vi "rsidr_core_global.vi"() -> ()   [LabVIEW 2020, in "Rohde&Schwarz RTx Oscilloscopes.lvlib"] (continued)
 is white. You can select another monochrome color, or a color scale.\n\nAvailable Repeated Capabilities:\nReferenceWfm: RW1, RW2, RW3, RW4\r\n\nRemote-control command(s):\nREFCurve<m>:WCOLor"}, {"Level"=2, "Class Only"=TRUE, "Identifier"="", "Descriptive Name"="Reference", "Data Type"=0, "Command"="", "Access"=0, "Range Table"="", "Read Callback"="", "Write Callback"="", "Supported Models"="", "Instrument Options"="", "Flags"=0, "Help"="Contains attributes for Reference settings."}, {"Level"=3, "Class Only"=FALSE, "Identifier"="RSRTX_ATTR_REFERENCE_WAVEFORM_SOURCE", "Descriptive Name"="Reference Waveform Source", "Data Type"=0, "Command"="REFC{ReferenceWfm}:SOUR", "Access"=2, "Range Table"="rsrtx_rngReferenceWaveformParameter", "Read Callback"="", "Write Callback"="", "Supported Models"="", "Instrument Options"="", "Flags"=0, "Help"="Selects the source waveform to be used as a reference.\n\nAvailable Repeated Capabilities:\nReferenceWfm: RW1, RW2, RW3, RW4\r\n\nRemote-control command(s):\nREFCurve<m>:SOURce"}, {"Level"=3, "Class Only"=FALSE, "Identifier"="RSRTX_ATTR_REFERENCE_WAVEFORM_UPDATE", "Descriptive Name"="Reference Waveform Update", "Data Type"=4, "Command"="REFC{ReferenceWfm}:UPD", "Access"=1, "Range Table"="", "Read Callback"="", "Write Callback"="", "Supported Models"="", "Instrument Options"="", "Flags"=0, "Help"="Copies the selected source waveform with all its settings to the memory of the reference waveform\n\nAvailable Repeated Capabilities:\nReferenceWfm: RW1, RW2, RW3, RW4\r\n\nRemote-control command(s):\nREFCurve<m>:UPDate"}, {"Level"=3, "Class Only"=FALSE, "Identifier"="RSRTX_ATTR_REFERENCE_WAVEFORM_DISPLAY_ENABLED", "Descriptive Name"="Reference Waveform Display Enabled", "Data Type"=3, "Command"="REFC{ReferenceWfm}:STAT", "Access"=2, "Range Table"="", "Read Callback"="", "Write Callback"="", "Supported Models"="", "Instrument Options"="", "Flags"=0, "Help"="If enabled, the reference waveform is displayed in the diagram.\n\nAvailable Repeated Capabilities:\nReferenceWfm: RW1, RW2, RW3, RW4\r\n\nRemote-control command(s):\nREFCurve<m>:STATe"}, {"Level"=3, "Class Only"=FALSE, "Identifier"="RSRTX_ATTR_REFERENCE_WAVEFORM_LOAD_FROM_FILE", "Descriptive Name"="Reference Waveform Load From File", "Data Type"=2, "Command"="REFC{ReferenceWfm}:LOAD", "Access"=1, "Range Table"="", "Read Callback"="", "Write Callback"="", "Supported Models"="", "Instrument Options"="", "Flags"=0, "Help"="Loads the waveform data from the indicated reference file to the reference storage. To load the instrument settings, use REFCurve<m>: LOAD: STATe.\n\nAvailable Repeated Capabilities:\nReferenceWfm: RW1, RW2, RW3, RW4\r\n\nRemote-control command(s):\nREFCurve<m>:LOAD"}, {"Level"=3, "Class Only"=FALSE, "Identifier"="RSRTX_ATTR_REFERENCE_WAVEFORM_LOAD_CONFIGURATION", "Descriptive Name"="Reference Waveform Load Configuration", "Data Type"=4, "Command"="REFC{ReferenceWfm}:LOAD:STAT", "Access"=1, "Range Table"="", "Read Callback"="", "Write Callback"="", "Supported Models"="", "Instrument Options"="", "Flags"=0, "Help"="Loads the instrument settings in addition to the reference waveform data. The waveform data must be loaded before the settings. The settings are only available if the file was stored to the internal storage /INT/REF ERENCE and never written to an external storage (USB stick).\n\nAvailable Repeated Capabilities:\nReferenceWfm: RW1, RW2, RW3, RW4\r\n\nRemote-control command(s):\nREFCurve<m>:LOAD:STATe"}, {"Level"=3, "Class Only"=FALSE, "Identifier"="RSRTX_ATTR_REFERENCE_WAVEFORM_SAVE_TO_FILE", "Descriptive Name"="Reference Waveform Save To File", "Data Type"=2, "Command"="REFC{ReferenceWfm}:SAVE", "Access"=1, "Range Table"="", "Read Callback"="", "Write Callback"="", "Supported Models"="", "Instrument Options"="", "Flags"=0, "Help"="Stores the reference waveform the specified file. For instrument model &apos;&apos; is parameter <FileName> ignored.\n\nAvailable Repeated Capabilities:\nReferenceWfm: RW1, RW2, RW3, RW4\r\n\nRemote-control command(s):\nREFCurve<m>:SAVE"}, {"Level"=3, "Class Only"=FALSE, "Identifier"="RSRTX_ATTR_REFERENCE_WAVEFORM_CATALOG", "Descriptive Name"="Reference Waveform Catalog", "Data Type"=2, "Command"="REFC{ReferenceWfm}:SOUR:CAT?", "Access"=0, "Range Table"="", "Read Callback"="", "Write Callback"="", "Supported Models"="", "Instrument Options"="", "Flags"=0, "Help"="Returns the source waveform - channel, math or reference waveform.\n\nAvailable Repeated Capabilities:\nReferenceWfm: RW1, RW2, RW3, RW4\r\n\nRemote-control command(s):\nREFCurve<m>:SOURce:CATalog?"}, {"Level"=2, "Class Only"=TRUE, "Identifier"="", "Descriptive Name"="Scaling", "Data Type"=0, "Command"="", "Access"=0, "Range Table"="", "Read Callback"="", "Write Callback"="", "Supported Models"="", "Instrument Options"="", "Flags"=0, "Help"="Contains attributes for Scalling settings."}, {"Level"=3, "Class Only"=FALSE, "Identifier"="RSRTX_ATTR_REFERENCE_WAVEFORM_VERTICAL_SCALE", "Descriptive Name"="Reference Waveform Vertical Scale", "Data Type"=1, "Command"="REFC{ReferenceWfm}:VERT:SCAL", "Access"=2, "Range Table"="", "Read Callback"="", "Write Callback"="", "Supported Models"="", "Instrument Options"="", "Flags"=0, "Help"="Sets the scale factor for the reference waveform if vertical scaling is set to Independent.\n\nAvailable Repeated Capabilities:\nReferenceWfm: RW1, RW2, RW3, RW4\r\n\nRemote-control command(s):\nREFCurve<m>:VERTical:SCALe"}, {"Level"=3, "Class Only"=FALSE, "Identifier"="RSRTX_ATTR_REFERENCE_WAVEFORM_VERTICAL_POSITION", "Descriptive Name"="Reference Waveform Vertical Position", "Data Type"=1, "Command"="REFC{ReferenceWfm}:VERT:POS", "Access"=2, "Range Table"="", "Read Callback"="", "Write Callback"="", "Supported Models"="", "Instrument Options"="", "Flags"=0, "Help"="Moves the reference waveform and its horizontal axis up or down in the diagram, if vertical scaling is set to Independent.\n\nAvailable Repeated Capabilities:\nReferenceWfm: RW1, RW2, RW3, RW4\r\n\nRemote-control command(s):\nREFCurve<m>:VERTical:POSition"}, {"Level"=3, "Class Only"=FALSE, "Identifier"="RSRTX_ATTR_REFERENCE_WAVEFORM_HORIZONTAL_SCALE", "Descriptive Name"="Reference Waveform Horizontal Scale", "Data Type"=1, "Command"="REFC{ReferenceWfm}:HOR:SCAL", "Access"=2, "Range Table"="", "Read Callback"="", "Write Callback"="", "Supported Models"="", "Instrument Options"="", "Flags"=0, "Help"="Changes the horizontal scale (timebase) of the reference waveform independent of the channel waveform settings.\n\nAvailable Repeated Capabilities:\nReferenceWfm: RW1, RW2, RW3, RW4\r\n\nRemote-control command(s):\nREFCurve<m>:HORizontal:SCALe"}, {"Level"=3, "Class Only"=FALSE, "Identifier"="RSRTX_ATTR_REFERENCE_WAVEFORM_HORIZONTAL_POSITION", "Descriptive Name"="Reference Waveform Horizontal Position", "Data Type"=1, "Command"="REFC{ReferenceWfm}:HOR:POS", "Access"=2, "Range Table"="", "Read Callback"="", "Write Callback"="", "Supported Models"="", "Instrument Options"="", "Flags"=0, "Help"="Changes the horizontal position of the reference waveform independent of the channel waveform settings.\n\nAvailable Repeated Capabilities:\nReferenceWfm: RW1, RW2, RW3, RW4\r\n\nRemote-control command(s):\nREFCurve<m>:HORizontal:POSition"}, {"Level"=1, "Class Only"=TRUE, "Identifier"="", "Descriptive Name"="Mask", "Data Type"=0, "Command"="", "Access"=0, "Range Table"="", "Read Callback"="", "Write Callback"="", "Supported Models"="", "Instrument Options"="", "Flags"=0, "Help"="Contains attributes for Masks settings."}, {"Level"=2, "Class Only"=FALSE, "Identifier"="RSRTX_ATTR_MASK_ENABLED", "Descriptive Name"="Mask Enabled", "Data Type"=3, "Command"="MASK:STAT", "Access"=2, "Range Table"="", "Read Callback"="", "Write Callback"="", "Supported Models"="", "Instrument Options"="", "Flags"=0, "Help"="Turns the mask test mode on or off. When turning off, any temporarily stored new masks are deleted.\n\nAvailable Repeated Capabilities:\nNone\n\nRemote-control command(s):\nMASK:STATe"}, {"Level"=2, "Class Only"=FALSE, "Identifier"="RSRTX_ATTR_MASK_SOURCE", "Descriptive Name"="Mask Source", "Data Type"=0, "Command"="MASK:SOUR", "Access"=2, "Range Table"="rsrtx_rngSource", "Read Callback"="", "Write Callback"="", "Supported Models"="", "Instrument Options"="", "Flags"=0, "Help"="Defines the channel to be compared with the mask.\n\nAvailable Repeated Capabilities:\nNone\n\nRemote-control command(s):\nMASK:SOURce"}, {"Level"=2, "Class Only"=FALSE, "Identifier"="RSRTX_ATTR_MASK_TEST", "Descriptive Name"="Mask Test", "Data Type"=0, "Command"="MASK:TEST", "Access"=2, "Range Table"="rsrtx_rngMaskCondition", "Read Callback"="", "Write Callback"="", "Supported Models"="", "Instrument Options"="", "Flags"=0, "Help"="Starts, finishes or interrupts a mask test.\n\nAvailable Repeated Capabilities:\nNone\n\nRemote-control command(s):\nMASK:TEST"}, {"Level"=2, "Class Only"=FALSE, "Identifier"="RSRTX_ATTR_MASK_COPY_CHANNEL", "Descriptive Name"="Mask Copy Channel", "Data Type"=4, "Command"="MASK:CHC", "Access"=1, "Range Table"="", "Read Callback"="", "Write Callback"="", "Supported Models"="", "Instrument Options"="", "Flags"=0, "Help"="Creates a mask from the envelope waveform of the test source set with MASK:SOURce.\n\nAvailable Repeated Capabilities:\nNone\n\nRemote-control command(s):\nMASK:CHCopy"}, {"Level"=2, "Class Only"=FALSE, "Identifier"="RSRTX_ATTR_MASK_HIT_COUNT", "Descriptive Name"="Mask Hit Count", "Data Type"=0, "Command"="MASK:VCO?", "Access"=0, "Range Table"="", "Read Callback"="", "Write Callback"="", "Supported Models"="", "Instrument Options"="", "Flags"=0, "Help"="Returns the number of acquistions that hit the mask.\n\nAvailable Repeated Capabilities:\nNone\n\nRemote-control command(s):\nMASK:VCOunt?"}, {"Level"=2, "Class Only"=FALSE, "Identifier"="RSRTX_ATTR_MASK_COUNT", "Descriptive Name"="Mask Count", "Data Type"=0, "Command"="MASK:COUN?", "Access"=0, "Range Table"="", "Read Callback"="", "Write Callback"="", "Supported Models"="", "Instrument Options"="", "Flags"=0, "Help"="Returns the number of tested acquisitions.\n\nAvailable Repeated Capabilities:\nNone\n\nRemote-control command(s):\nMASK:COUNt?"}, {"Level"=2, "Class Only"=FALSE, "Identifier"="RSRTX_ATTR_MASK_SEGMENT_CAPTURE_MODE", "Descriptive Name"="Mask Segment Capture Mode", "Data Type"=0, "Command"="MASK:CAPT", "Access"=2, "Range Table"="RsRtx_rngMaskCaptureMode", "Read Callback"="", "Write Callback"="", "Supported Models"="", "Instrument Options"="K15", "Flags"=0, "Help"="Only available with history. Selects whether all acquisitions are stored in segments, or only failed acquisition. You can use the history to analyze the segments.\n\nAvailable Repeated Capabilities:\nNone\n\nRemote-control command(s):\nMASK:CAPTure[:MODE]"}, {"Level"=2, "Class Only"=FALSE, "Identifier"="RSRTX_ATTR_MASK_STORE", "Descriptive Name"="Mask Store", "Data Type"=2, "Command"="MASK:SAVE", "Access"=1, "Range Table"="", "Read Callback"="", "Write Callback"="", "Supported Models"="", "Instrument Options"="", "Flags"=0, "Help"="Saves the current mask in the specified file.\n\nAvailable Repeated Capabilities:\nNone\n\nRemote-control command(s):\nMASK:SAVE"}, {"Level"=2, "Class Only"=FALSE, "Identifier"="RSRTX_ATTR_MASK_LOAD", "Descriptive Name"="Mask Load", "Data Type"=2, "Command"="MASK:LOAD", "Access"=1, "Range Table"="", "Read Callback"="", "Write Callback"="", "Supported Models"="", "Instrument Options"="", "Flags"=0, "Help"="Loads a stored mask from the specified file.\n\nAvailable Repeated Capabilities:\nNone\n\nRemote-control command(s):\nMASK:LOAD"}, {"Level"=2, "Class Only"=FALSE, "Identifier"="RSRTX_ATTR_MASK_TEST_ACTION_BEEP", "Descriptive Name"="Mask Test Action Beep", "Data Type"=0, "Command"="MASK:ACT:SOUN:EVEN:MODE", "Access"=2, "Range Table"="rsrtx_rngMaskTestActionExecution", "Read Callback"="", "Write Callback"="", "Supported Models"="", "Instrument Options"="", "Flags"=0, "Help"="Sets when and how often the generates a beep sound will be executed.\n\nAvailable Repeated Capabilities:\nNone\n\nRemote-control command(s):\nMASK:ACTion:SOUNd:EVENt:MODE"}, {"Level"=2, "Class Only"=FALSE, "Identifier"="RSRTX_ATTR_MASK_TEST_ACTION_STOP", "Descriptive Name"="Mask Test Action Stop", "Data Type"=0, "Command"="MASK:ACT:STOP:EVEN:MODE", "Access"=2, "Range Table"="rsrtx_rngMaskTestActionExecution", "Read Callback"="", "Write Callback"="", "Supported Models"="", "Instrument Options"="", "Flags"=0, "Help"="Sets when and how often the stops the waveform acquisition. will be executed.\n\nAvailable Repeated Capabilities:\nNone\n\nRemote-control command(s):\nMASK:ACTion:STOP:EVENt:MODE"}, {"Level"=2, "Class Only"=FALSE, "Identifier"="RSRTX_ATTR_MASK_TEST_ACTION_SCREENSHOT", "Descriptive Name"="Mask Test Action Screenshot", "Data Type"=0, "Command"="MASK:ACT:SCRS:EVEN:MODE", "Access"=2, "Range Table"="rsrtx_rngMaskTestActionExecution", "Read Callback"="", "Write Callback"="", "Supported Models"="", "Instrument Options"="", "Flags"=0, "Help"="Sets when and how often the saves a screenshot according to printer output settings will be executed.\n\nAvailable Repeated Capabilities:\nNone\n\nRemote-control command(s):\nMASK:ACTion:SCRSave:EVENt:MODE"}, {"Level"=2, "Class Only"=FALSE, "Identifier"="RSRTX_ATTR_MASK_TEST_ACTION_SCREENSHOT_DESTINATION", "Descriptive Name"="Mask Test Action Screenshot Destination", "Data Type"=2, "Command"="MASK:ACT:SCRS:DEST", "Access"=2, "Range Table"="", "Read Callback"="", "Write Callback"="", "Supported Models"="", "Instrument Options"="", "Flags"=0, "Help"="Defines the path and filename for a screenshot that will be saved on mask violation. The file format is PNG, the filename is incremented automatically.\n\nAvailable Repeated Capabilities:\nNone\n\nRemote-control command(s):\nMASK:ACTion:SCRSave:DESTination"}, {"Level"=2, "Class Only"=FALSE, "Identifier"="RSRTX_ATTR_MASK_TEST_ACTION_SAVES_WAVEFORM", "Descriptive Name"="Mask Test Action Saves Waveform", "Data Type"=0, "Command"="MASK:ACT:WFMSave:EVEN:MODE", "Access"=2, "Range Table"="rsrtx_rngMaskTestActionExecution", "Read Callback"="", "Write Callback"="", "Supported Models"="", "Instrument Options"="", "Flags"=0, "Help"="Sets when and how often the saves the waveform data according to the screenshot output settings will be executed.\n\nAvailable Repeated Capabilities:\nNone\n\nRemote-control command(s):\nMASK:ACTion:WFMSave:EVENt:MODE"}, {"Level"=2, "Class Only"=FALSE, "Identifier"="RSRTX_ATTR_MASK_TEST_ACTION_SAVES_WAVEFORM_DESTINATION", "Descriptive Name"="Mask Test Action Saves Waveform Destination", "Data Type"=2, "Command"="MASK:ACT:WFMS:DEST", "Access"=2, "Range Table"="", "Read Callback"="", "Write Callback"="", "Supported Models"="", "Instrument Options"="", "Flags"=0, "Help"="Defines the path and filename for a waveform data that will be saved on mask violation. The file format is CSV, the filename is incremented automatically.\n\nAvailable Repeated Capabilities:\nNone\n\nRemote-control command(s):\nMASK:ACTion:WFMSave:DESTination"}, {"Level"=2, "Class Only"=FALSE, "Identifier"="RSRTX_ATTR_MASK_TEST_ACTION_PULSE", "Descriptive Name"="Mask Test Action Pulse", "Data Type"=0, "Command"="MASK:ACT:PULS:EVEN:MODE", "Access"=2, "Range Table"="rsrtx_rngMaskTestActionExecution", "Read Callback"="", "Write Callback"="", "Supported Models"="", "Instrument Options"="", "Flags"=0, "Help"="Creates a trigger out pulse on mask violation.\n\nAvailable Repeated Capabilities:\nNone\n\nRemote-control command(s):\nMASK:ACTion:PULSe:EVENt:MODE"}, {"Level"=2, "Class Only"=FALSE, "Identifier"="RSRTX_ATTR_MASK_TEST_ACTION_AUX_OUTPUT_ENABLED", "Descriptive Name"="Mask Test Action AUX Output Enabled", "Data Type"=3, "Command"="MASK:ACT:YOUT:ENAB", "Access"=2, "Range Table"="", "Read Callback"="", "Write Callback"="", "Supported Models"="", "Instrument Options"="", "Flags"=0, "Help"="Creates a pulse on the AUX OUT connector if the mask is violated. This selection sets the configuration of the AUX OUT connector to Mask Violation.\n\nAvailable Repeated Capabilities:\nNone\n\nRemote-control command(s):\nMASK:ACTion:YOUT:ENABle"}, {"Level"=2, "Class Only"=FALSE, "Identifier"="RSRTX_ATTR_MASK_TEST_VIOLATION_COUNT_BEEP", "Descriptive Name"="Mask Test Violation Count Beep", "Data Type"=0, "Command"="MASK:ACT:SOUN:EVEN:COUN", "Access"=2, "Range Table"="", "Read Callback"="", "Write Callback"="", "Supported Models"="", "Instrument Options"="", "Flags"=0, "Help"="Sets the number of mask violations after which the generates a beep sound is executed.\n\nAvailable Repeated Capabilities:\nNone\n\nRemote-control command(s):\nMASK:ACTion:SOUNd:EVENt:COUNt"}, {"Level"=2, "Class Only"=FALSE, "Identifier"="RSRTX_ATTR_MASK_TEST_VIOLATION_COUNT_STOP", "Descriptive Name"="Mask Test Violation Count Stop", "Data Type"=0, "Command"="MASK:ACT:STOP:EVEN:COUN", "Access"=2, "Range Table"="", "Read Callback"="", "Write Callback"="", "Supported Models"="", "Instrument Options"="", "Flags"=0, "Help"="Sets the number of mask violations after which the stops the waveform acquisition is executed.\n\nAvailable Repeated Capabilities:\nNone\n\nRemote-control command(s):\nMASK:ACTion:STOP:EVENt:COUNt"}, {"Level"=2, "Class Only"=FALSE, "Identifier"="RSRTX_ATTR_MASK_TEST_VIOLATION_COUNT_SCREENSHOT", "Descriptive Name"="Mask Test Violation Count Screenshot", "Data Type"=0, "Command"="MASK:ACT:SCRS:EVEN:COUN", "Access"=2, "Range Table"="", "Read Callback"="", "Write Callback"="", "Supported Models"="", "Instrument Options"="", "Flags"=0, "Help"="Sets the number of mask violations after which the saves a screenshot according to printer output settings is executed.\n\nAvailable Repeated Capabilities:\nNone\n\nRemote-control command(s):\nMASK:ACTion:SCRSave:EVENt:COUNt"}, {"Level"=2, "Class Only"=FALSE, "Identifier"="RSRTX_ATTR_MASK_TEST_VIOLATION_COUNT_PRINT", "Descriptive Name"="Mask Test Violation Count Print", "Data Type"=0, "Command"="MASK:ACT:PRIN:EVEN:COUN", "Access"=2, "Range Table"="", "Read Callback"="", "Write Callback"="", "Supported Models"="", "Instrument Options"="", "Flags"=0, "Help"="Sets the number of mask violations after which the prints a screenshot to a printer connected to the USB connector on the front or rear panel is executed.\n\nAvailable Repeated Capabilities:\nNone\n\nRemote-control command(s):\nMASK:ACTion:PRINt:EVENt:COUNt"}, {"Level"=2, "Class Only"=FALSE, "Identifier"="RSRTX_ATTR_MASK_TEST_VIOLATION_COUNT_SAVES_WAVEFORM", "Descriptive Name"="Mask Test Violation Count Saves Waveform", "Data Type"=0, "Command"="MASK:ACT:WFMS:EVEN:COUN", "Access"=2, "Range Table"="", "Read Callback"="", "Write Callback"="", "Supported Models"="", "Instrument Options"="", "Flags"=0, "Help"="Sets the number of mask violations after which the saves the waveform data according to the screenshot output settings is executed.\n\nAvailable Repeated Capabilities:\nNone\n\nRemote-control command(s):\nMASK:ACTion:WFMSave:EVENt:COUNt"}, {"Level"=2, "Class Only"=FALSE, "Identifier"="RSRTX_ATTR_MASK_TEST_VIOLATION_COUNT_PULSE", "Descriptive Name"="Mask Test Violation Count Pulse", "Data Type"=0, "Command"="MASK:ACT:PULS:EVEN:COUN", "Access"=2, "Range Table"="", "Read Callback"="", "Write Callback"="", "Supported Models"="", "Instrument Options"="", "Flags"=0, "Help"="Sets the number of mask violations after which the action is executed.\n\nAvailable Repeated Capabilities:\nNone\n\nRemote-control command(s):\nMASK:ACTion:PULSe:EVENt:COUNt"}, {"Level"=2, "Class Only"=FALSE, "Identifier"="RSRTX_ATTR_MASK_TEST_VIOLATION_PULSE_LENGTH", "Descriptive Name"="Mask Test Violation Pulse Length", "Data Type"=1, "Command"="MASK:ACT:PULS:PLEN", "Access"=2, "Range Table"="", "Read Callback"="", "Write Callback"="", "Supported Models"="", "Instrument Options"="", "Flags"=0, "Help"="Sets the pulse width of the trigger out pulse that is created on mask violation.\n\nAvailable Repeated Capabilities:\nNone\n\nRemote-control command(s):\nMASK:ACTion:PULSe:PLENgth"}, {"Level"=2, "Class Only"=FALSE, "Identifier"="RSRTX_ATTR_MASK_TEST_VIOLATION_PULSE_POLARITY", "Descriptive Name"="Mask Test Violation Pulse Polarity", "Data Type"=0, "Command"="MASK:ACT:PULS:POL", "Access"=2, "Range Table"="rsrtx_rngPolarity", "Read Callback"="", "Write Callback"="", "Supported Models"="", "Instrument Options"="", "Flags"=0, "Help"="Sets the polarity of the trigger out pulse that is created on mask violation.\n\nAvailable Repeated Capabilities:\nNone\n\nRemote-control command(s):\nMASK:ACTion:PULSe:POLarity"}, {"Level"=2, "Class Only"=FALSE, "Identifier"="RSRTX_ATTR_MASK_RESET_TEST_COUNTER", "Descriptive Name"="Mask Reset Test Counter", "Data Type"=4, "Command"="MASK:RES:COUN", "Access"=1, "Range Table"="", "Read Callback"="", "Write Callback"="", "Supported Models"="", "Instrument Options"="", "Flags"=0, "Help"="Sets the counters of passed and failed acquisitions to Zero.\n\nAvailable Repeated Capabilities:\nNone\n\nRemote-control command(s):\nMASK:RESet:COUNter"}, {"Level"=2, "Class Only"=TRUE, "Identifier"="", "Descriptive Name"="Mask Scaling", "Data Type"=0, "Command"="", "Access"=0, "Range Table"="", "Read Callback"="", "Write Callback"="", "Supported Models"="", "Instrument Options"="", "Flags"=0, "Help"="Contains attributes for Mask Scalling settings."}, {"Level"=3, "Class Only"=FALSE, "Identifier"="RSRTX_ATTR_MASK_VERTICAL_OFFSET", "Descriptive Name"="Mask Vertical Offset", "Data Type"=1, "Command"="MASK:YPOS", "Access"=2, "Range Table"="", "Read Callback"="", "Write Callback"="", "Supported Models"="", "Instrument Options"="", "Flags"=0, "Help"="Moves the mask vertically within the display.\n\nAvailable Repeated Capabilities:\nNone\n\nRemote-control command(s):\nMASK:YPOSition"}, {"Level"=3, "Class Only"=FALSE, "Identifier"="RSRTX_ATTR_MASK_VERTICAL_SCALING", "Descriptive Name"="Mask Vertical Scaling", "Data Type"=1, "Command"="MASK:YSC", "Access"=2, "Range Table"="", "Read Callback"="", "Write Callback"="", "Supported Models"="", "Instrument Options"="", "Flags"=0, "Help"="Changes the vertical scaling to stretch or compress the mask in y-direction.\n\nAvailable Repeated Capabilities:\nNone\n\nRemote-control command(s):\nMASK:YSCale"}, {"Level"=3, "Class Only"=FALSE, "Identifier"="RSRTX_ATTR_MASK_VERTICAL_WIDTH", "Descriptive Name"="Mask Vertical Width", "Data Type"=1, "Command"="MASK:YWID", "Access"=2, "Range Table"="", "Read Callback"="", "Write Callback"="", "Supported Models"="", "Instrument Options"="", "Flags"=0, "Help"="Changes the width of the mask in vertical direction.\n\nAvailable Repeated Capabilities:\nNone\n\nRemote-control command(s):\nMASK:YWIDth"}, {"Level"=3, "Class Only"=FALSE, "Identifier"="RSRTX_ATTR_MASK_HORIZONTAL_WIDTH", "Descriptive Name"="Mask Horizontal Width", "Data Type"=1, "Command"="MASK:XWID", "Access"=2, "Range Table"="", "Read Callback"="", "Write Callback"="", "Supported Models"="", "Instrument Options"="", "Flags"=0, "Help"="Changes the width of the mask in horizontal direction.\n\nAvailable Repeated Capabilities:\nNone\n\nRemote-control command(s):\nMASK:XWIDth"}, {"Level"=1, "Class Only"=TRUE, "Identifier"="", "Descriptive Name"="Search", "Data Type"=0, "Command"="", "Access"=0, "Range Table"="", "Read Callback"="", "Write Callback"="", "Supported Models"="", "Instrument Options"="", "Flags"=0, "Help"="Contains attributes for searching functions."}, {"Level"=2, "Class Only"=FALSE, "Identifier"="RSRTX_ATTR_SEARCH_ENABLED", "Descriptive Name"="Search Enabled", "Data Type"=3, "Command"="SEAR:STAT", "Access"=2, "Range Table"="", "Read Callback"="", "Write Callback"="", "Supported Models"="", "Instrument Options"="", "Flags"=0, "Help"="Enables and disables the search mode.\n\nAvailable Repeated Capabilities:\nNone\n\nRemote-control command(s):\nSEARch:STATe"}, {"Level"=2, "Class Only"=FALSE, "Identifier"="RSRTX_ATTR_SEARCH_CONDITION", "Descriptive Name"="Search Condition", "Data Type"=0, "Command"="SEAR:COND", "Access"=2, "Range Table"="rsrtx_rngSearchCondition", "Read Callback"="", "Write Callback"="", "Supported Models"="", "Instrument Options"="", "Flags"=0, "Help"="Selects the symptom you want to search for.\n\nAvailable Repeated Capabilities:\nNone\n\nRemote-control command(s):\nSEARch:CONDition"}, {"Level"=2, "Class Only"=FALSE, "Identifier"="RSRTX_ATTR_SEARCH_SOURCE", "Descriptive Name"="Search Source", "Data Type"=0, "Command"="SEAR:SOUR", "Access"=2, "Range Table"="rsrtx_rngSearchSource", "Read Callback"="", "Write Callback"="", "Supported Models"="", "Instrument Options"="", "Flags"=0, "Help"="Selects the waveform to be analyzed. One of the active channel, math, and reference waveforms can be searched.\n\nAvailable Repeated Capabilities:\nNone\n\nRemote-control command(s):\nSEARch:SOURce"}, {"Level"=2, "Class Only"=FALSE, "Identifier"="RSRTX_ATTR_SEARCH_TRIGGER_EDGE_SLOPE", "Descriptive Name"="Search Trigger Edge Slope", "Data Type"=0, "Command"="SEAR:TRIG:EDGE:SLOP", "Access"=2, "Range Table"="rsrtx_rngSearchSlope", "Read Callback"="", "Write Callback"="", "Supported Models"="", "Instrument Options"="", "Flags"=0, "Help"="Sets the slope to be found.\n\nAvailable Repeated Capabilities:\nNone\n\nRemote-control command(s):\nSEARch:TRIGger:EDGE:SLOPe"}, {"Level"=2, "Class Only"=FALSE, "Identifier"="RSRTX_ATTR_SEARCH_TRIGGER_EDGE_LEVEL", "Descriptive Name"="Search Trigger Edge Level", "Data Type"=1, "Command"="SEAR:TRIG:EDGE:LEV", "Access"=2, "Range Table"="", "Read Callback"="", "Write Callback"="", "Supported Models"="", "Instrument Options"="", "Flags"=0, "Help"="Sets the voltage level for the edge search.\n\nAvailable Repeated Capabilities:\nNone\n\nRemote-control command(s):\nSEARch:TRIGger:EDGE:LEVel"}, {"Level"=2, "Class Only"=FALSE, "Identifier"="RSRTX_ATTR_SEARCH_TRIGGER_EDGE_HYSTERSIS", "Descriptive Name"="Search Trigger Edge Hystersis", "Data Type"=1, "Command"="SEAR:TRIG:EDGE:LEV:DELT", "Access"=2, "Range Table"="", "Read Callback"="", "Write Callback"="", "Supported Models"="", "Instrument Options"="", "Flags"=0, "Help"="Sets a hysteresis range above and below the search level to avoid unwanted search results caused by noise oscillation around the level.\n\nAvailable Repeated Capabilities:\nNone\n\nRemote-control command(s):\nSEARch:TRIGger:EDGE:LEVel:DELTa"}, {"Level"=2, "Class Only"=FALSE, "Identifier"="RSRTX_ATTR_SEARCH_TRIGGER_WIDTH_LEVEL", "Descriptive Name"="Search Trigger Width Level", "Data Type"=1, "Command"="SEAR:TRIG:WIDT:LEV", "Access"=2, "Range Table"="", "Read Callback"="", "Write Callback"="", "Supported Models"="", "Instrument Options"="", "Flags"=0, "Help"="Sets the voltage level on which the pulse width is measured.\n\nAvailable Repeated Capabilities:\nNone\n\nRemote-control command(s):\nSEARch:TRIGger:WIDTh:LEVel"}, {"Level"=2, "Class Only"=FALSE, "Identifier"="RSRTX_ATTR_SEARCH_TRIGGER_WIDTH_HYSTERSIS", "Descriptive Name"="Search Trigger Width Hystersis", "Data Type"=1, "Command"="SEAR:TRIG:WIDT:LEV:DELT", "Access"=2, "Range Table"="", "Read Callback"="", "Write Callback"="", "Supported Models"="", "Instrument Options"="", "Flags"=0, "Help"="Defines a range around the width value.\n\nAvailable Repeated Capabilities:\nNone\n\nRemote-control command(s):\nSEARch:TRIGger:WIDTh:LEVel:DELTa"}, {"Level"=2, "Class Only"=FALSE, "Identifier"="RSRTX_ATTR_SEARCH_TRIGGER_WIDTH_WIDTH", "Descriptive Name"="Search Trigger Width Width", "Data Type"=1, "Command"="SEAR:TRIG:WIDT:WIDT", "Access"=2, "Range Table"="", "Read Callback"="", "Write Callback"="", "Supported Models"="", "Instrument Options"="", "Flags"=0, "Help"="Sets the reference pulse width, the nominal value for comparisons.\n\nAvailable Repeated Capabilities:\nNone\n\nRemote-control command(s):\nSEARch:TRIGger:WIDTh:WIDTh"}, {"Level"=2, "Class Only"=FALSE, "Identifier"="RSRTX_ATTR_SEARCH_TRIGGER_WIDTH_DELTA", "Descriptive Name"="Search Trigger Width Delta", "Data Type"=1, "Command"="SEAR:TRIG:WIDT:DELT", "Access"=2, "Range Table"="", "Read Callback"="", "Write Callback"="", "Supported Models"="", "Instrument Options"="", "Flags"=0, "Help"="Sets a range delta t to the reference pulse width.\n\nAvailable Repeated Capabilities:\nNone\n\nRemote-control command(s):\nSEARch:TRIGger:WIDTh:DELTa"}, {"Level"=2, "Class Only"=FALSE, "Identifier"="RSRTX_ATTR_SEARCH_TRIGGER_WIDTH_POLARITY", "Descriptive Name"="Search Trigger Width Polarity", "Data Type"=0, "Command"="SEAR:TRIG:WIDT:POL", "Access"=2, "Range Table"="rsrtx_rngPolarity", "Read Callback"="", "Write Callback"="", "Supported Models"="", "Instrument Options"="", "Flags"=0, "Help"="Sets the polarity of the pulse.\n\nAvailable Repeated Capabilities:\nNone\n\nRemote-control command(s):\nSEARch:TRIGger:WIDTh:POLarity"}, {"Level"=2, "Class Only"=FALSE, "Identifier"="RSRTX_ATTR_SEARCH_TRIGGER_WIDTH_RANGE", "Descriptive Name"="Search Trigger Width Range", "Data Type"=0, "Command"="SEAR:TRIG:WIDT:RANG", "Access"=2, "Range Table"="rsrtx_rngSearchRange", "Read Callback"="", "Write Callback"="", "Supported Models"="", "Instrument Options"="", "Flags"=0, "Help"="Sets how the measured pulse width is compared with the given limit(s).\n\nAvailable Repeated Capabilities:\nNone\n\nRemote-control command(s):\nSEARch:TRIGger:WIDTh:RANGe"}, {"Level"=2, "Class Only"=FALSE, "Identifier"="RSRTX_ATTR_SEARCH_TRIGGER_PEAK_POLARITY", "Descriptive Name"="Search Trigger Peak Polarity", "Data Type"=0, "Command"="SEAR:MEAS:PEAK:POL", "Access"=2, "Range Table"="rsrtx_rngSearchSlope", "Read Callback"="", "Write Callback"="", "Supported Models"="", "Instrument Options"="", "Flags"=0, "Help"="Indicates the polarity of a the pulse to be searched for a peak.\n\nAvailable Repeated Capabilities:\nNone\n\nRemote-control command(s):\nSEARch:MEASure:PEAK:POLarity"}, {"Level"=2, "Class Only"=FALSE, "Identifier"="RSRTX_ATTR_SEARCH_TRIGGER_PEAK_LIMIT", "Descriptive Name"="Search Trigger Peak Limit", "Data Type"=1, "Command"="SEAR:MEAS:LEV:PEAK:MAGN", "Access"=2, "Range Table"="", "Read Callback"="", "Write Callback"="", "Supported Models"="", "Instrument Options"="", "Flags"=0, "Help"="Sets the voltage level for the edge search.\n\nAvailable Repeated Capabilities:\nNone\n\nRemote-control command(s):\nSEARch:MEASure:LEVel:PEAK:MAGNitude"}, {"Level"=2, "Class Only"=FALSE, "Identifier"="RSRTX_ATTR_SEARCH_TRIGGER_RISE_TIME_POLARITY", "Descriptive Name"="Search Trigger Rise Time Polarity", "Data Type"=0, "Command"="SEAR:TRIG:RIS:SLOP", "Access"=2, "Range Table"="rsrtx_rngSearchSlope", "Read Callback"="", "Write Callback"="", "Supported Models"="", "Instrument Options"="", "Flags"=0, "Help"="Sets the slope to be found.\n\nAvailable Repeated Capabilities:\nNone\n\nRemote-control command(s):\nSEARch:TRIGger:RISetime:SLOPe"}, {"Level"=2, "Class Only"=FALSE, "Identifier"="RSRTX_ATTR_SEARCH_TRIGGER_RISE_TIME_LEVEL_LOWER", "Descriptive Name"="Search Trigger Rise Time Level Lower", "Data Type"=1, "Command"="SEAR:TRIG:LEV:RIS:LOW", "Access"=2, "Range Table"="", "Read Callback"="", "Write Callback"="", "Supported Models"="", "Instrument Options"="", "Flags"=0, "Help"="Sets the voltage threshold. When the signal crosses this level, the rise time measurement starts or stops depending on the selected slope.\n\nAvailable Repeated Capabilities:\nNone\n\nRemote-control command(s):\nSEARch:TRIGger:LEVel:RISetime:LOWer"}, {"Level"=2, "Class Only"=FALSE, "Identifier"="RSRTX_ATTR_SEARCH_TRIGGER_RISE_TIME_LEVEL_UPPER", "Descriptive Name"="Search Trigger Rise Time Level Upper", "Data Type"=1, "Command"="SEAR:TRIG:LEV:RIS:UPP", "Access"=2, "Range Table"="", "Read Callback"="", "Write Callback"="", "Supported Models"="", "Instrument Options"="", "Flags"=0, "Help"="Sets the voltage threshold. When the signal crosses this level, the rise time measurement starts or stops depending on the selected slope.\n\nAvailable Repeated Capabilities:\nNone\n\nRemote-control command(s):\nSEARch:TRIGger:LEVel:RISetime:UPPer"}, {"Level"=2, "Class Only"=FALSE, "Identifier"="RSRTX_ATTR_SEARCH_TRIGGER_RISE_TIME_RANGE", "Descriptive Name"="Search Trigger Rise Time Range", "Data Type"=0, "Command"="SEAR:TRIG:RIS:RANG", "Access"=2, "Range Table"="rsrtx_rngSearchRange", "Read Callback"="", "Write Callback"="", "Supported Models"="", "Instrument Options"="", "Flags"=0, "Help"="Sets how the measured rise or fall time is compared with the given limit(s).\n\nAvailable Repeated Capabilities:\nNone\n\nRemote-control command(s):\nSEARch:TRIGger:RISetime:RANGe"}, {"Level"=2, "Class Only"=FALSE, "Identifier"="RSRTX_ATTR_SEARCH_TRIGGER_RISE_TIME_REFERENCE_TIME", "Descriptive Name"="Search Trigger Rise Time Reference Time", "Data Type"=1, "Command"="SEAR:TRIG:RIS:TIME", "Access"=2, "Range Table"="", "Read Callback"="", "Write Callback"="", "Supported Models"="", "Instrument Options"="", "Flags"=0, "Help"="Sets the reference rise or fall time, the nominal value for comparisons.\n\nAvailable Repeated Capabilities:\nNone\n\nRemote-control command(s):\nSEARch:TRIGger:RISetime:TIME"}, {"Level"=2, "Class Only"=FALSE, "Identifier"="RSRTX_ATTR_SEARCH_TRIGGER_RISE_TIME_DELTA_TIME", "Descriptive Name"="Search Trigger Rise Time Delta Time", "Data Type"=1, "Command"="SEAR:TRIG:RIS:DELT", "Access"=2, "Range Table"="", "Read Callback"="", "Write Callback"="", "Supported Models"="", "Instrument Options"="", "Flags"=0, "Help"="Sets a range delta t to the reference rise/fall time set with Time if Range is set to Within or Outside.\n\nAvailable Repeated Capabilities:\nNone\n\nRemote-control command(s):\nSEARch:TRIGger:RISetime:DELTa"}, {"Level"=2, "Class Only"=FALSE, "Identifier"="RSRTX_ATTR_SEARCH_TRIGGER_RUNT_POLARITY", "Descriptive Name"="Search Trigger Runt Polarity", "Data Type"=0, "Command"="SEAR:TRIG:RUNT:POL", "Access"=2, "Range Table"="rsrtx_rngSearchSlope", "Read Callback"="", "Write Callback"="", "Supported Models"="", "Instrument Options"="", "Flags"=0, "Help"="Indicates the polarity of a the runt to be searched for.\n\nAvailable Repeated Capabilities:\nNone\n\nRemote-control command(s):\nSEARch:TRIGger:RUNT:POLarity"}, {"Level"=2, "Class Only"=FALSE, "Identifier"="RSRTX_ATTR_SEARCH_TRIGGER_RUNT_LEVEL_LOWER", "Descriptive Name"="Search Trigger Runt Level Lower", "Data Type"=1, "Command"="SEAR:TRIG:LEV:RUNT:LOW", "Access"=2, "Range Table"="", "Read Callback"="", "Write Callback"="", "Supported Models"="", "Instrument Options"="", "Flags"=0, "Help"="Sets the lower|upper voltage threshold for runt detection. A positive runt crosses the lower level twice without crossing the lower|upper level.\n\nAvailable Repeated Capabilities:\nNone\n\nRemote-control command(s):\nSEARch:TRIGger:LEVel:RUNT:LOWer"}, {"Level"=2, "Class Only"=FALSE, "Identifier"="RSRTX_ATTR_SEARCH_TRIGGER_RUNT_LEVEL_UPPER", "Descriptive Name"="Search Trigger Runt Level Upper", "Data Type"=1, "Command"="SEAR:TRIG:LEV:RUNT:UPPer", "Access"=2, "Range Table"="", "Read Callback"="", "Write Callback"="", "Supported Models"="", "Instrument Options"="", "Flags"=0, "Help"="Sets the lower|upper voltage threshold for runt detection. A positive runt crosses the lower level twice without crossing the lower|upper level.\n\nAvailable Repeated Capabilities:\nNone\n\nRemote-control command(s):\nSEARch:TRIGger:LEVel:RUNT:UPPer"}, {"Level"=2, "Class Only"=FALSE, "Identifier"="RSRTX_ATTR_SEARCH_TRIGGER_RUNT_RANGE", "Descriptive Name"="Search Trigger Runt Range", "Data Type"=0, "Command"="SEAR:TRIG:RUNT:RANG", "Access"=2, "Range Table"="rsrtx_rngSearchRange", "Read Callback"="", "Write Callback"="", "Supported Models"="", "Instrument Options"="", "Flags"=0, "Help"="Sets how the measured pulse width is compared with the given limit(s).\n\nAvailable Repeated Capabilities:\nNone\n\nRemote-control command(s):\nSEARch:TRIGger:RUNT:RANGe"}, {"Level"=2, "Class Only"=FALSE, "Identifier"="RSRTX_ATTR_SEARCH_TRIGGER_RUNT_WIDTH", "Descriptive Name"="Search Trigger Runt Width", "Data Type"=1, "Command"="SEAR:TRIG:RUNT:WIDT", "Access"=2, "Range Table"="", "Read Callback"="", "Write Callback"="", "Supported Models"="", "Instrument Options"="", "Flags"=0, "Help"="Configures the conditions for the runt trigger search.\n\nAvailable Repeated Capabilities:\nNone\n\nRemote-control command(s):\nSEARch:TRIGger:RUNT:WIDTh"}, {"Level"=2, "Class Only"=FALSE, "Identifier"="RSRTX_ATTR_SEARCH_TRIGGER_RUNT_DELTA_WIDTH", "Descriptive Name"="Search Trigger Runt Delta Width", "Data Type"=1, "Command"="SEAR:TRIG:RUNT:DELT", "Access"=2, "Range Table"="", "Read Callback"="", "Write Callback"="", "Supported Models"="", "Instrument Options"="", "Flags"=0, "Help"="Sets a range delta t to the reference rise/fall time set with Width if Range is set to Within or Outside.\n\nAvailable Repeated Capabilities:\nNone\n\nRemote-control command(s):\nSEARch:TRIGger:RUNT:DELTa"}, {"Level"=2, "Class Only"=FALSE, "Identifier"="RSRTX_ATTR_SEARCH_TRIGGER_D2C_CLOCK_SOURCE", "Descriptive Name"="Search Trigger Data2Clock Clock Source", "Data Type"=0, "Command"="SEAR:TRIG:DAT:CSO", "Access"=2, "Range Table"="rsrtx_rngSearchSource", "Read Callback"="", "Write Callback"="", "Supported Models"="", "Instrument Options"="", "Flags"=0, "Help"="Sets the waveform sourece for clock line. For setting waveform source of data line use RSRTX_ATTR_SEARCH_SOURCE.\n\nAvailable Repeated Capabilities:\nNone\n\nRemote-control command(s):\nSEARch:TRIGger:DATatoclock:CSOurce"}, {"Level"=2, "Class Only"=FALSE, "Identifier"="RSRTX_ATTR_SEARCH_TRIGGER_D2C_CLOCK_LEVEL", "Descriptive Name"="Search Trigger Data2Clock Clock Level", "Data Type"=1, "Command"="SEAR:TRIG:DAT:CLEV", "Access"=2, "Range Table"="", "Read Callback"="", "Write Callback"="", "Supported Models"="", "Instrument Options"="", "Flags"=0, "Help"="Sets the voltage levels for clock signals. Clock level and clock edge define the reference point for setup and hold time.\n\nAvailable Repeated Capabilities:\nNone\n\nRemote-control command(s):\nSEARch:TRIGger:DATatoclock:CLEVel"}, {"Level"=2, "Class Only"=FALSE, "Identifier"="RSRTX_ATTR_SEARCH_TRIGGER_D2C_DATA_LEVEL", "Descriptive Name"="Search Trigger Data2Clock Data Level", "Data Type"=1, "Command"="SEAR:TRIG:DAT:DLEV", "Access"=2, "Range Table"="", "Read Callback"="", "Write Callback"="", "Supported Models"="", "Instrument Options"="", "Flags"=0, "Help"="Sets the voltage levels for  data signals. The data level defines the point of data transition.\n\nAvailable Repeated Capabilities:\nNone\n\nRemote-control command(s):\nSEARch:TRIGger:DATatoclock:DLEVel"}, {"Level"=2, "Class Only"=FALSE, "Identifier"="RSRTX_ATTR_SEARCH_TRIGGER_D2C_CLOCK_HYSTERESIS", "Descriptive Name"="Search Trigger Data2Clock Clock Hysteresis", "Data Type"=1, "Command"="SEAR:TRIG:DAT:CLEV:DELT", "Access"=2, "Range Table"="", "Read Callback"="", "Write Callback"="", "Supported Models"="", "Instrument Options"="", "Flags"=0, "Help"="Sets a hysteresis range to the clock or data levels in order to avoid unwanted search results caused by noise oscillation around the level. For a rising edge, the hysteresis is below the search level. Otherwise, for a falling edge the hysteresis is above the level.\n\nAvailable Repeated Capabilities:\nNone\n\nRemote-control command(s):\nSEARch:TRIGger:DATatoclock:CLEVel:DELTa"}, {"Level"=2, "Class Only"=FALSE, "Identifier"="RSRTX_ATTR_SEARCH_TRIGGER_D2C_DATA_HYSTERESIS", "Descriptive Name"="Search Trigger Data2Clock Data Hysteresis", "Data Type"=1, "Command"="SEAR:TRIG:DAT:DLEV:DELT", "Access"=2, "Range Table"="", "Read Callback"="", "Write Callback"="", "Supported Models"="", "Instrument Options"="", "Flags"=0, "Help"="Sets a hysteresis range to the clock or data levels in order to avoid unwanted search results caused by noise oscillation around the level. For a rising edge, the hysteresis is below the search level. Otherwise, for a falling edge the hysteresis is above the level.\n\nAvailable Repeated Capabilities:\nNone\n\nRemote-control command(s):\nSEARch:TRIGger:DATatoclock:DLEVel:DELTa"}, {"Level"=2, "Class Only"=FALSE, "Identifier"="RSRTX_ATTR_SEARCH_TRIGGER_D2C_POLARITY", "Descriptive Name"="Search Trigger Data2Clock Polarity", "Data Type"=0, "Command"="SEAR:TRIG:DAT:CEDG", "Access"=2, "Range Table"="rsrtx_rngSearchSlope", "Read Callback"="", 
